vi "Transition Measurements.vi"   [LabVIEW 2020, in "NI_MAPro.lvlib"]
doc: "Accepts an input signal of a single waveform or an array of waveforms and measures the transition duration (rise or fall time), slew rate, undershoot, and overshoot of a selected positive or negative transition in each waveform. Wire data to the <B>signal in</B> input to determine the polymorphic instance to use or manually select the instance."
uses:
  NI_MAPro.lvlib
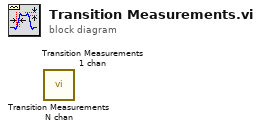
[diagram p0: block diagram]
diagram:
  n1 = call "Transition Measurements N chan.vi"() -> ()  [unwired: 6 in, 6 out]
  n2 = call "Transition Measurements 1 chan.vi"() -> ()  [unwired: 6 in, 6 out]
